vi "lead-lag_ctrl.vi"(6 "Mode":T1=enum."Tustin (Bilinear)", 8 "Sampling Time":dbl, 9 "tau":dbl, 10 "alpha":dbl, 11 "Input":dbl) -> (0 "Sampling\nTime Out":dbl, 3 "Output":dbl)   [LabVIEW 2018, in "DiscreteControllers.lvlib"]
doc: "Lead/Lag controller \nImplements (alpha*tau*s+1)/(tau*s+1) in discrete form.\nalpha > 1 (lead), alpha < 1 (lag)\nSelect the appropriate discretization mode."
uses:
  DiscreteControllers.lvlib
  TF_diff_mode.ctl
panel:
  in  "Initialize?":bool
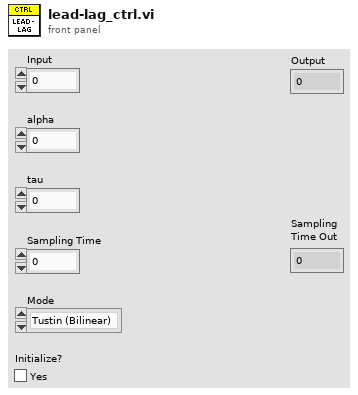
[diagram p1: front panel]
types:
  T1 = typedef "DiscreteControllers.lvlib/TF_diff_mode.ctl" = enum16{"Forward Euler", "Backward Euler", "Tustin (Bilinear)"}
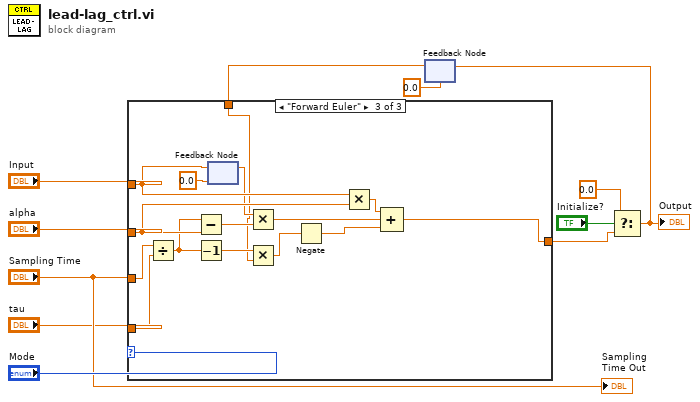
[diagram p0: block diagram]
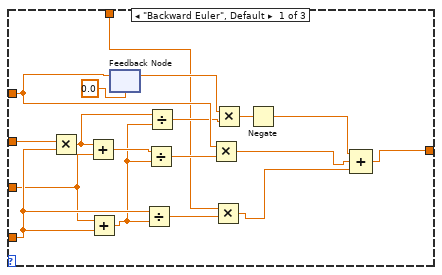
[diagram p2: hidden frame]
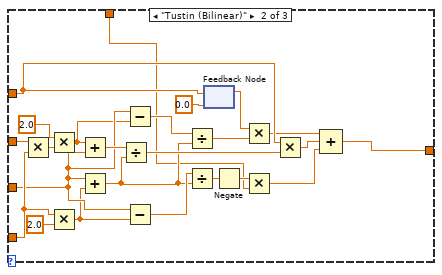
[diagram p3: hidden frame]
diagram:
  n1 = feedback #1(0.0) -> (w5:dbl)
  n2 = case shown="\"Forward Euler\"" "Mode" {
    tunnel: "Input" -> [w23 w45 w66]
    tunnel: "alpha" -> [w28 w53 w64]
    tunnel: "Sampling Time" -> [w13 w41 w68]
    tunnel: "tau" -> [w27 w52 w67]
    tunnel: [w14 w35 w58] -> w3
    tunnel: w5 -> [w12 w30 w54]
    frame "Backward Euler", Default {
      n3 = Multiply(x=w28, y=w27) -> (x*y=w22:dbl)
      n4 = Add(x=w22, y=w13) -> (x+y=w25:dbl)
      n5 = Add(x=w13, y=w27) -> (x+y=w21:dbl)
      n6 = feedback #2(0.0 ("Input")) -> (w19:dbl)
      n7 = feedback-in #2(w23) -> ()
      n8 = Divide(x=w27, y=w21) -> (x/y=w26:dbl)
      n9 = Divide(x=w25, y=w21) -> (x/y=w24:dbl)
      n10 = Divide(x=w22, y=w21) -> (x/y=w20:dbl)
      n11 = Multiply(x=w23, y=w24) -> (x*y=w16:dbl)
      n12 = Multiply(x=w12, y=w26) -> (x*y=w15:dbl)
      n13 = Multiply(x=w19, y=w20) -> (x*y=w18:dbl)
      n14 = Negate(x=w18) -> (-x=w17:dbl)
      n15 = Compound Arithmetic op=ADD(w17, w16, w15) -> (w14:dbl)
    }
    frame "Tustin (Bilinear)" {
      n16 = Multiply(x=w53, y=w52) -> (x*y=w47:dbl)
      n17 = Multiply(x=2.0, y=w47) -> (x*y=w34:dbl)
      n18 = Multiply(x=w52, y=2.0) -> (x*y=w40:dbl)
      n19 = Add(x=w34, y=w41) -> (x+y=w50:dbl)
      n20 = Add(x=w41, y=w40) -> (x+y=w38:dbl)
      n21 = Divide(x=w50, y=w38) -> (x/y=w49:dbl)
      n22 = Subtract(x=w41, y=w34) -> (x-y=w48:dbl)
      n23 = Subtract(x=w41, y=w40) -> (x-y=w39:dbl)
      n24 = Divide(x=w48, y=w38) -> (x/y=w43:dbl)
      n25 = Divide(x=w39, y=w38) -> (x/y=w33:dbl)
      n26 = feedback-in #3(w45) -> ()
      n27 = feedback #3(0.0 ("Input")) -> (w42:dbl)
      n28 = Negate(x=w33) -> (-x=w32:dbl)
      n29 = Multiply(x=w42, y=w43) -> (x*y=w37:dbl)
      n30 = Multiply(x=w32, y=w30) -> (x*y=w31:dbl)
      n31 = Multiply(x=w45, y=w49) -> (x*y=w36:dbl)
      n32 = Compound Arithmetic op=ADD(w37, w36, w31) -> (w35:dbl)
    }
    frame "Forward Euler" {
      n33 = Divide(x=w68, y=w67) -> (x/y=w61:dbl)
      n34 = Subtract(x=w61, y=w64) -> (x-y=w63:dbl)
      n35 = Decrement(x=w61) -> (x-1=w60:dbl)
      n36 = feedback-in #4(w66) -> ()
      n37 = feedback #4(0.0 ("Input")) -> (w62:dbl)
      n38 = Multiply(x=w62, y=w63) -> (x*y=w57:dbl)
      n39 = Multiply(x=w60, y=w54) -> (x*y=w59:dbl)
      n40 = Negate(x=w59) -> (-x=w56:dbl)
      n41 = Multiply(x=w66, y=w64) -> (x*y=w55:dbl)
      n42 = Compound Arithmetic op=ADD(w55, w57, w56) -> (w58:dbl)
    }
  }
  n43 = Select(t=0.0, s="Initialize?", f=w3) -> (s? t:f=w2:dbl)
  "Output" <- w2
  n44 = feedback-in #1(w2) -> ()
  "Sampling\nTime Out" <- "Sampling Time"
